vi "Initialize.vi"(7 "Serial Configuration":T1={"Baud Rate"=9600, "Parity"=0, "Data Bits"=8, "Stop Bits"=10, "Flow Control"=0} {"Flow Control" items=["None", "XON/XOFF", "RTS/CTS", "XON/XOFF & RTS/CTS", "DTR/DSR", "XON/XOFF & DTR/DSR"]; "Stop Bits" items=["1.0"=10, "1.5"=15, "2.0"=20]; "Data Bits" items=["7"=7, "8"=8]; "Parity" items=["None", "Odd", "Even", "Mark", "Space"]; "Baud Rate" items=["300"=300, "600"=600, "1200"=1200, "2400"=2400, "4800"=4800, "9600"=9600, "19200"=19200]}, 8 "error in (no error)":errorcluster, 9 "Reset (True)":bool=TRUE, 10 "ID Query (True)":bool=TRUE, 11 "VISA resource name":refnum<visa-resource-name>) -> (0 "error out":errorcluster, 3 "VISA resource name out":refnum<visa-resource-name>)   [LabVIEW 2020, in "Keithley 2600 Series.lvlib"]
doc: "Establishes communication with the instrument and optionally performs an instrument identification query and/or an instrument reset. It also places the instrument in a default state needed for other instrument driver operations. Therefore, call this VI before calling other instrument driver VIs for this instrument. Generally, you need to call the <b>Initialize</b> VI only once at the beginning of an application."
uses:
  Keithley 2600 Series.lvlib
panel:
  # "(c) 2020 National Instruments.  ALL RIGHTS RESERVED."
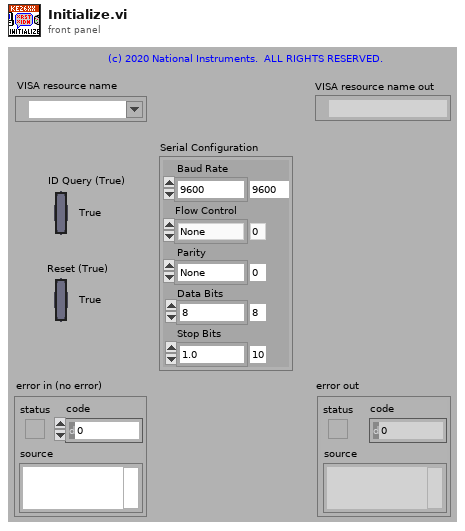
[diagram p1: front panel]
types:
  T1 = cluster{"Baud Rate":u32, "Parity":u16, "Data Bits":u16, "Stop Bits":u16, "Flow Control":u16}
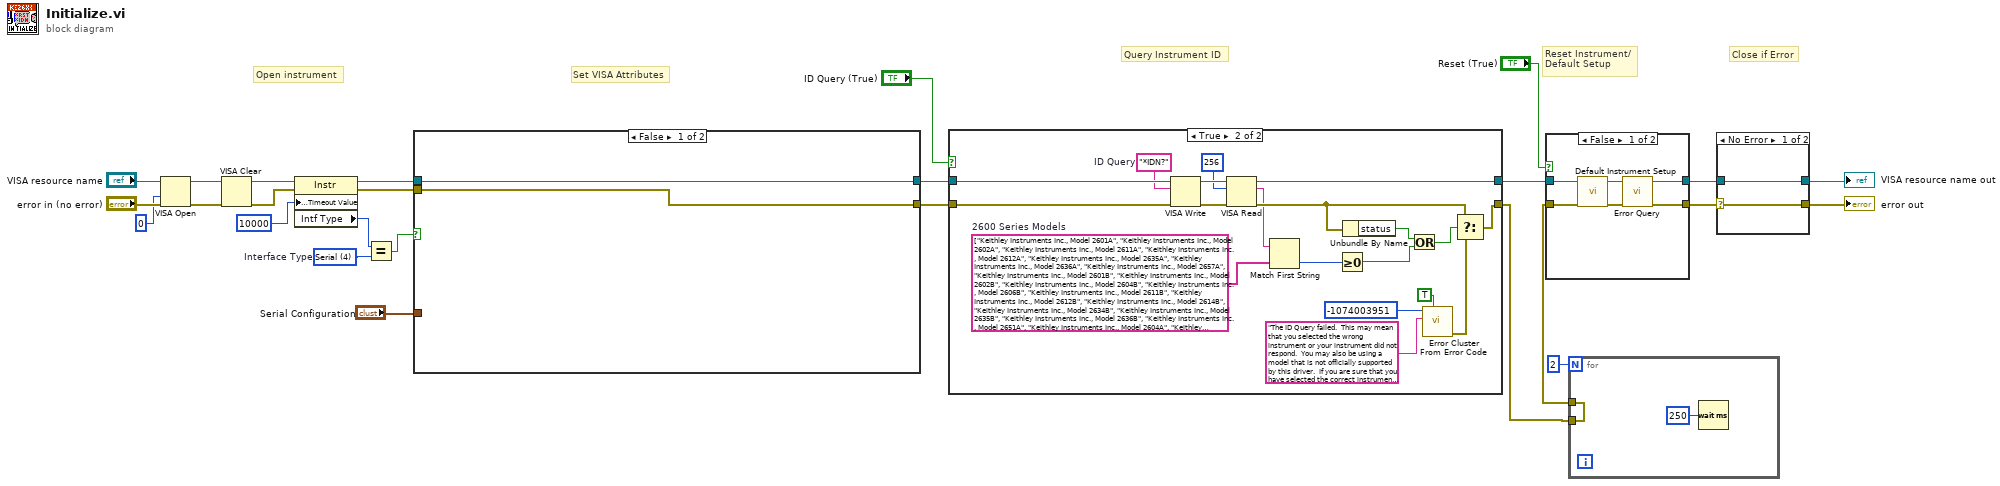
[diagram p0: block diagram]
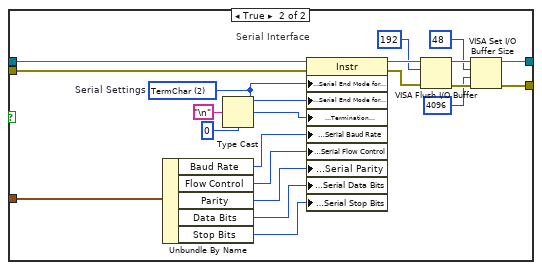
[diagram p2: hidden frame]
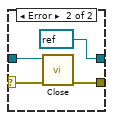
[diagram p3: hidden frame]
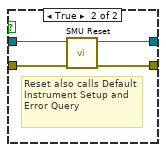
[diagram p4: hidden frame]
diagram:
  w11 = u16 4 items=["GPIB"=1, "VXI"=2, "GPIB-VXI"=3, "Serial"=4, "PXI"=5, "TCPIP"=6, "USB"=7]  # Interface Type
  # "Set VISA Attributes"
  # "Close if Error"
  # "Query Instrument ID"
  # "Reset Instrument/\nDefault Setup"
  # "Open instrument"
  n1 = VISA Open(access mode=u32 0, error in (no error)="error in (no error)", VISA resource name="VISA resource name") -> (VISA resource name=w19:refnum<visa-resource-name>, error out=w18:errorcluster)  [unwired: 2 in]
  n2 = VISA Clear(VISA resource name=w19, error in (no error)=w18) -> (VISA resource name out=w17:refnum<visa-resource-name>, error out=w16:errorcluster)
  n3 = property class="Instr"(reference=w17, error in=w16, "General Settings:Timeout Value"=u32 10000) -> (reference out=w9:refnum<visa-resource-name>, error out=w8:errorcluster, "Intf Type"=w10:u16)
  n4 = Equal?(x=w10, y=w11) -> (x = y?=w5:bool)
  n5 = case shown="False" w5 {
    tunnel: [w27 w46] -> w7
    tunnel: [w28 w43] -> w6
    tunnel: w9 -> [w27 w48]
    tunnel: w8 -> [w28 w49]
    tunnel: "Serial Configuration" -> [_ w29]
    frame False {
    }
    frame True {
      w36 = u16 2 items=["None", "LastBit", "TermChar"]  # Serial Settings
      # "Serial Interface"
      n6 = Unbundle By Name(w29) -> ("Baud Rate"=w34:u32, "Flow Control"=w31:u16, "Parity"=w32:u16, "Data Bits"=w33:u16, "Stop Bits"=w30:u16)
      n7 = Type Cast(type=u8 0, x="\n" ("Line Feed Constant")) -> (*(type *) &x=w35:u8)
      n8 = property class="Instr"(reference=w48, error in=w49, "Serial Settings:Serial End Mode for Reads"=w36, "Serial Settings:Serial End Mode for Writes"=w36, "Message Based Settings:Termination Character"=w35, "Serial Settings:Serial Baud Rate"=w34, "Serial Settings:Serial Flow Control"=w31, "Serial Settings:Serial Parity"=w32, "Serial Settings:Serial Data Bits"=w33, "Serial Settings:Serial Stop Bits"=w30) -> (reference out=w42:refnum<visa-resource-name>, error out=w45:errorcluster)
      n9 = VISA Flush I/O Buffer(VISA resource name=w42, mask (16)=u16 192, error in (no error)=w45) -> (VISA resource name out=w47:refnum<visa-resource-name>, error out=w44:errorcluster)
      n10 = VISA Set I/O Buffer Size(VISA resource name=w47, mask (16)=u16 48, size (4096)=u32 4096 ("size (0)"), error in (no error)=w44) -> (VISA resource name out=w46:refnum<visa-resource-name>, error out=w43:errorcluster)
    }
  }
  n11 = case shown="True" "ID Query (True)" {
    tunnel: [w50 w70] -> w2
    tunnel: [w51 w67] -> w26
    tunnel: w7 -> [w51 w68]
    tunnel: w6 -> [w50 w69]
    frame False {
    }
    frame True {
      w53 = string[] ["Keithley Instruments Inc., Model 2601A", "Keithley Instruments Inc., Model 2602A", "Keithley Instruments Inc., Model 2611A", "Keithley Instruments Inc., Model 2612A", "Keithley Instruments Inc., Model 2635A", "Keithley Instruments Inc., Model 2636A", "Keithley Instruments Inc., Model 2657A", "Keithley Instruments Inc., Model 2601B", "Keithley Instruments Inc., Model 2602B", "Keithley Instruments Inc., Model 2604B", "Keithley Instruments Inc., Model 2606B", "Keithley Instruments Inc., Model 2611B", "Keithley Instruments Inc., Model 2612B", "Keithley Instruments Inc., Model 2614B", "Keithley Instruments Inc., Model 2634B", "Keithley Instruments Inc., Model 2635B", "Keithley Instruments Inc., Model 2636B", "Keithley Instruments Inc., Model 2651A", "Keithley Instruments Inc., Model 2604A", "Keithley Instruments Inc., Model 2614A", "Keithley Instruments Inc., Model 2634A", "Keithley Instruments, Model 2601B-PULSE"]  # 2600 Series Models
      w63 = "*IDN?"  # ID Query
      n12 = VISA Write(VISA resource name=w68, write buffer=w63, error in (no error)=w69) -> (VISA resource name out=w66:refnum<visa-resource-name>, error out=w65:errorcluster)  [unwired: 1 out]
      n13 = VISA Read(VISA resource name=w66, byte count=u32 256, error in (no error)=w65) -> (VISA resource name out=w67:refnum<visa-resource-name>, read buffer=w52:string, error out=w58:errorcluster)  [unwired: 1 out]
      n14 = Match First String(2:w53, 3:w52) -> (0:w54:i32)  [unwired: 1 out]
      n15 = Greater Or Equal To 0?(x=w54) -> (x >= 0?=w56:bool)
      n16 = Unbundle By Name(w58) -> ("status"=w57:bool)
      n17 = Or(x=w57, y=w56) -> (x .or. y?=w55:bool)
      n18 = call <vilib>:"Error Cluster From Error Code.vi"("show call chain? (False)"=TRUE, "error message (\"\")"="The ID Query failed.  This may mean that you selected the wrong instrument or your instrument did not respond.  You may also be using a model that is not officially supported by this driver.  If you are sure that you have selected the correct instrument and it is responding, try disabling the ID Query." ("Source (VI Name)"), "error code (0)"=-1074003951 ("Code")) -> ("error out"=w62:errorcluster)  [unwired: 6 in]
      n19 = Select(t=w58, s=w55, f=w62) -> (s? t:f=w70:errorcluster)
    }
  }
  n20 = for {
    N: 2 -> [_]
    tunnel: w2 -> [w71]
    tunnel: [w71] -> w1
    n21 = Wait (ms)(milliseconds to wait=u32 250) -> ()  [unwired: 1 out]
  }
  n22 = case shown="False" "Reset (True)" {
    tunnel: w1 -> [w77 w80]
    tunnel: [w74 w79] -> w12
    tunnel: w26 -> [w78 w82]
    tunnel: [w75 w81] -> w13
    frame False {
      n23 = call "Default Instrument Setup.vi"("error in (no error)"=w77, "VISA resource name"=w78) -> ("error out"=w73:errorcluster, "VISA resource name out"=w76:refnum<visa-resource-name>)  [unwired: 8 in]
      n24 = call "Error Query.vi"("error in (no error)"=w73, "VISA resource name"=w76) -> ("error out"=w74:errorcluster, "VISA resource name out"=w75:refnum<visa-resource-name>)  [unwired: 6 in, 2 out]
    }
    frame True {
      # "Reset also calls Default Instrument Setup and Error Query"
      n25 = call "SMU Reset.vi"("error in (no error)"=w80, "VISA resource name"=w82) -> ("error out"=w79:errorcluster, "VISA resource name out"=w81:refnum<visa-resource-name>)  [unwired: 8 in]
    }
  }
  n26 = case shown="No Error" w12 {
    selector: w12 -> [w83 w86]
    tunnel: w13 -> [w84 w87]
    tunnel: [w84 refnum<visa-resource-name> refnum ("VISA resource name out")] -> w15
    tunnel: [w83 w88] -> w14
    frame No Error {
    }
    frame Error {
      n27 = call "Close.vi"("error in (no error)"=w86, "VISA resource name"=w87) -> ("error out"=w88:errorcluster)  [unwired: 9 in]
    }
  }
  "VISA resource name out" <- w15
  "error out" <- w14
